vi "CleanUp.vi"(0 "object in":refnum<class "STP Protocol.lvclass">, 5 "error in (no error)":errorcluster) -> (14 "object out":refnum<class "STP Protocol.lvclass">, 19 "error out":errorcluster)   [LabVIEW 2023, in "HardwareAbstractionLayer_LVOOP.lvlib" / "CAN Application Protocols Lib.lvlib" / "STP Protocol.lvclass"]
uses:
  STP Protocol.lvclass
  STP Protocol.lvclass/STP Protocol.ctl
  CAN Lib/NI-XNET_class/NI-XNET.lvclass
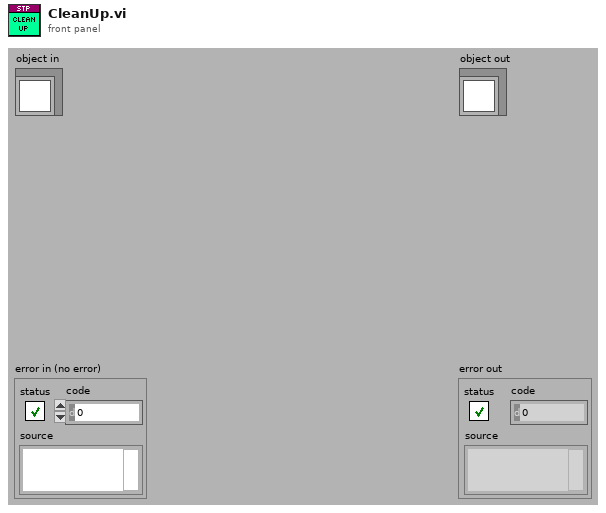
[diagram p1: front panel]
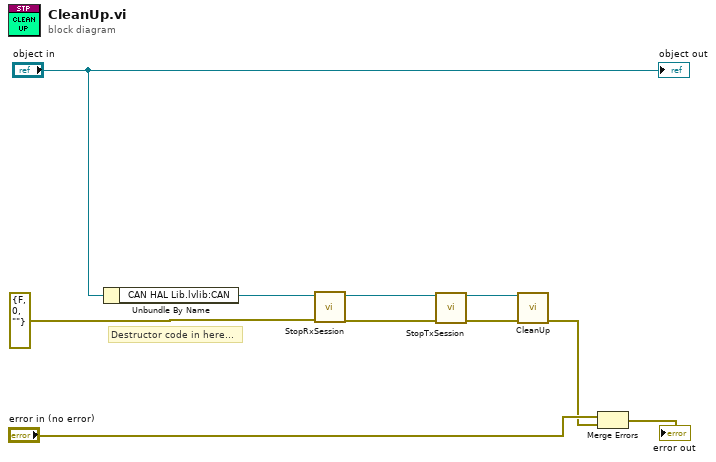
[diagram p0: block diagram]
diagram:
  # "Destructor code in here..."
  n1 = Unbundle By Name("object in") -> ("CAN HAL Lib.lvlib:CAN"=w6:refnum<class "NI-XNET.lvclass">)
  n2 = call-dynamic "StopRxSession.vi"("error in (no error)"=errorcluster {"status"=FALSE, "code"=0, "source"=""}, "NI-XNET in"=w6) -> ("error out"=w3:errorcluster, "NI-XNET out"=w4:refnum<class "NI-XNET.lvclass">)  [unwired: 8 in]
  n3 = call-dynamic "StopTxSession.vi"("error in (no error)"=w3, "NI-XNET in"=w4) -> ("error out"=w2:errorcluster, "NI-XNET out"=w1:refnum<class "NI-XNET.lvclass">)  [unwired: 8 in]
  n4 = call-dynamic "CleanUp.vi"("object in"=w1, "error in (no error)"=w2) -> ("error out"=w8:errorcluster)  [unwired: 12 in, 1 out]
  n5 = Merge Errors("error in (no error)", w8) -> (→"error out":errorcluster)
  "object out" <- "object in"
